vi "Run.vi"(8 "error in (no error)":errorcluster caption="entrée d'erreur (pas d'erreur)", 11 "20newsgroups.lvclass":refnum<class "20newsgroups.lvclass">) -> (0 "error out":errorcluster caption="sortie d'erreur", 2 "Data":string, 3 "20newsgroups.lvclass 2":refnum<class "20newsgroups.lvclass">)   [LabVIEW 2020, in "20newsgroups.lvclass"]
doc: "Returns :\n\n- data : list, length [n_samples]\nThe data list to learn.\n\n- target : array, shape [n_samples]\nThe target labels."
uses:
  20newsgroups.lvclass
  20newsgroups.lvclass/20newsgroups.ctl
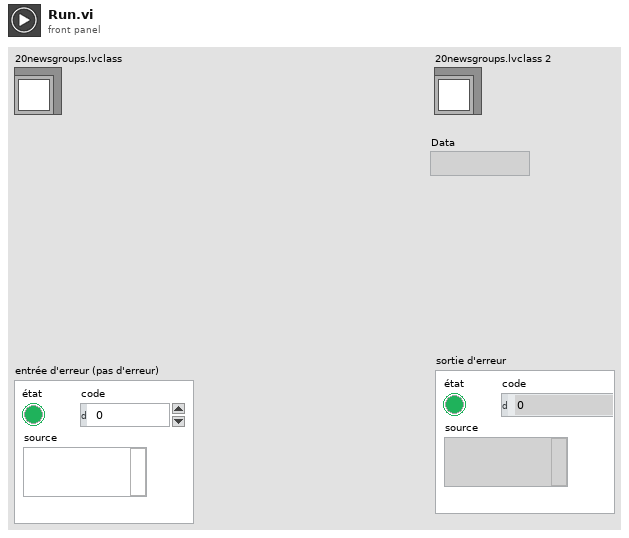
[diagram p1: front panel]
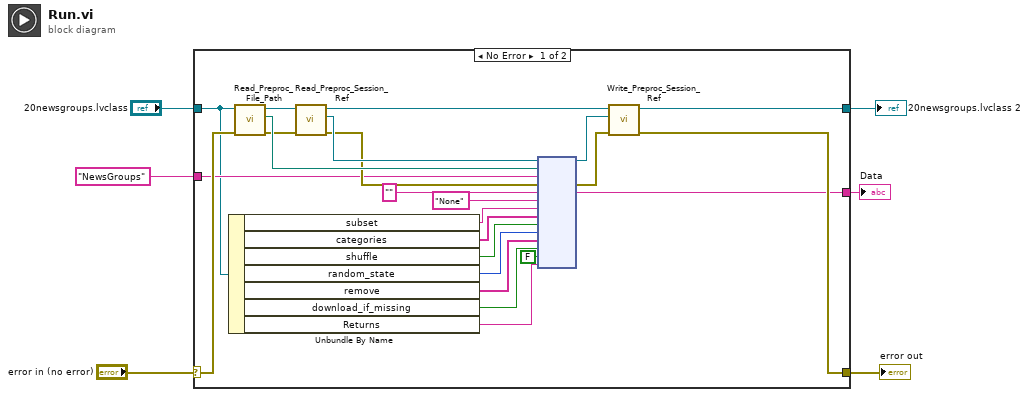
[diagram p0: block diagram]
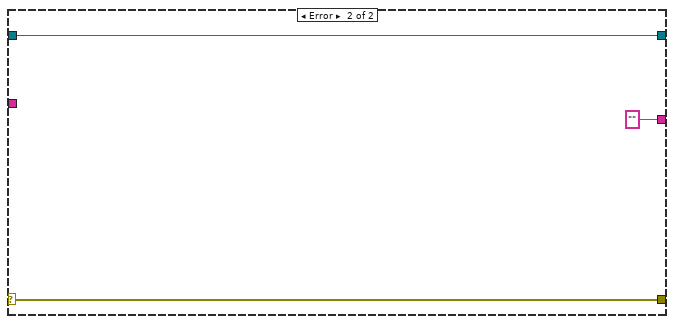
[diagram p2: hidden frame]
diagram:
  n1 = case shown="No Error" "error in (no error)" {
    selector: "error in (no error)" -> [w20 w33]
    tunnel: [w21 w33] -> w5
    tunnel: [w7 w32] -> w2
    tunnel: "20newsgroups.lvclass" -> [w10 w32]
    tunnel: "NewsGroups" -> [w19 _]
    tunnel: [w8 ""] -> w1
    frame No Error {
      n2 = Unbundle By Name(w10) -> ("subset"=w18:string, "categories"=w17:string[], "shuffle"=w15:bool, "random_state"=w14:i32, "remove"=w13:string[], "download_if_missing"=w12:bool, "Returns"=w9:string)
      n3 = call-dynamic "Read_Preproc_File_Path.vi"("error in (no error)"=w20, "Python in"=w10) -> ("error out"=w25:errorcluster, "File_Path"=w28:path, "Python out"=w30:refnum<class "20newsgroups.lvclass">)  [unwired: 7 in]
      n4 = call-dynamic "Read_Preproc_Session_Ref.vi"("error in (no error)"=w25, "Python in"=w30) -> ("error out"=w26:errorcluster, "Session_ref"=w27:refnum<k35>, "Python out"=w29:refnum<class "20newsgroups.lvclass">)  [unwired: 7 in]
      n5 = node(w27, w28, w19, w26, "", "None", w18, w17, w15, w14, w13, w12, FALSE, w9) -> (w22:refnum<k35>, w24:errorcluster, w8:string)  [unwired: 9 in, 2 out]
      n6 = call-dynamic "Write_Preproc_Session_Ref.vi"("error in (no error)"=w24, "Session_ref"=w22, "Python in"=w29) -> ("error out"=w21:errorcluster, "Python out"=w7:refnum<class "20newsgroups.lvclass">)  [unwired: 7 in]
    }
    frame Error {
    }
  }
  "error out" <- w5
  "20newsgroups.lvclass 2" <- w2
  "Data" <- w1
